vi "trasmision-datos-python-to-Labview.vi"() -> ()   [LabVIEW 2024]
panel:
  in  "trasmitir_START":bool
  in  "Server Closed":string="The server VI closed the connection."
  in  "Stop":bool
  out "Biosignal Graph":dbl[](graph)
  out "*(type *) &x":dbl[](array[numeric])
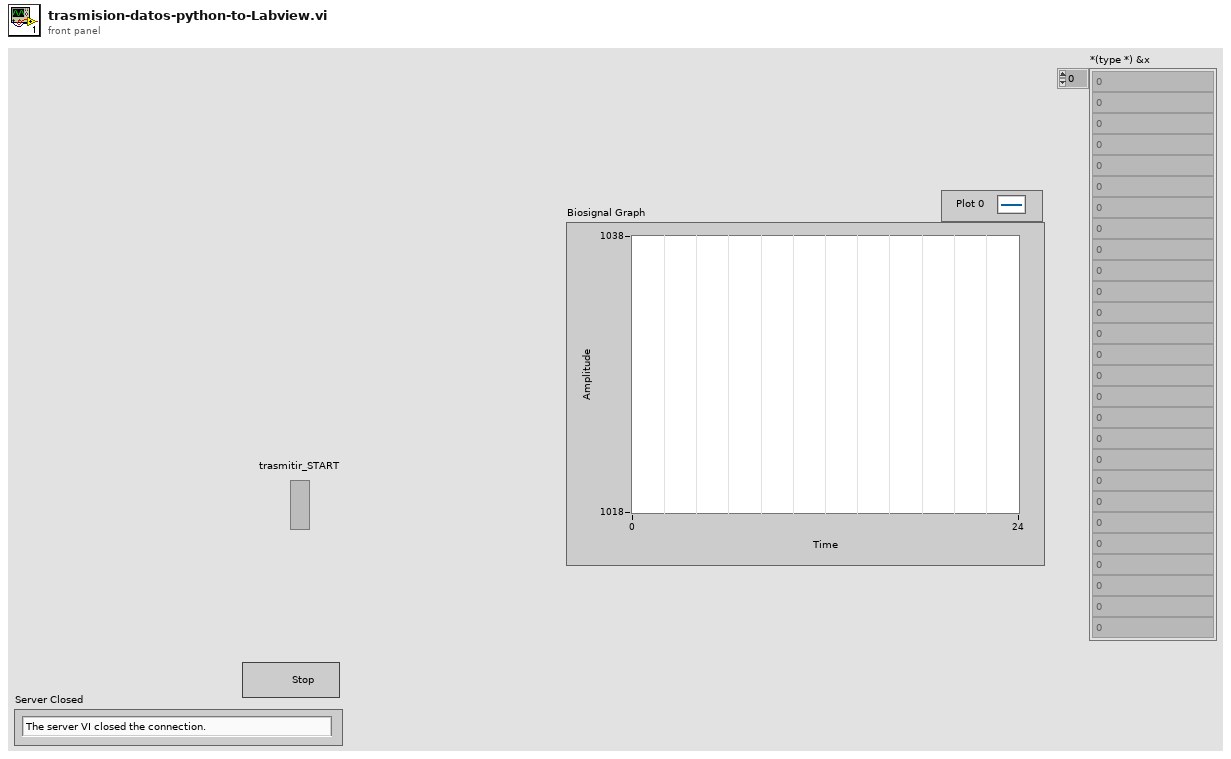
[diagram p1: front panel]
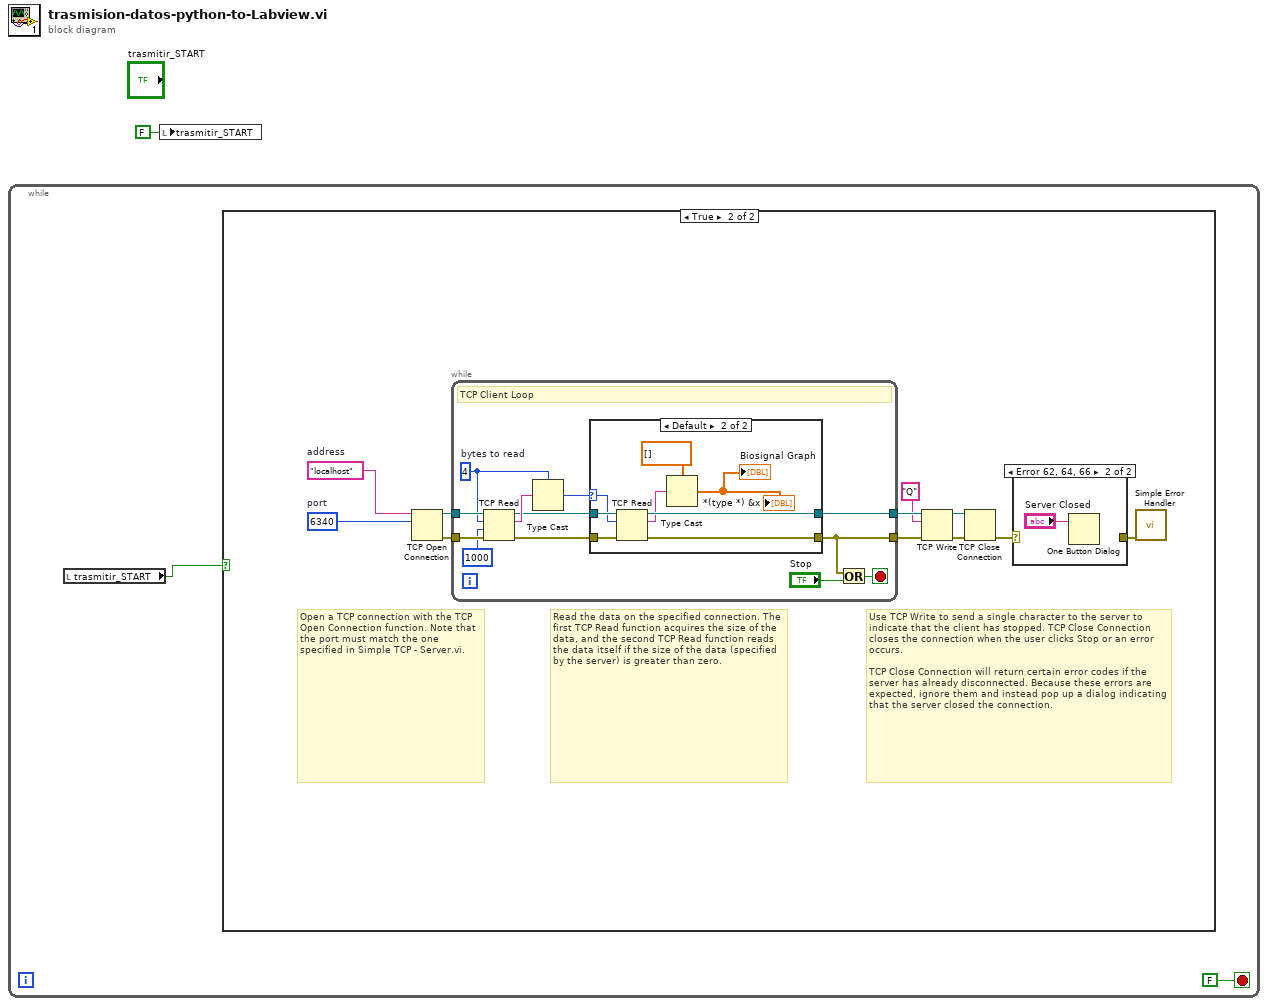
[diagram p0: block diagram]
diagram:
  n1 = while {
    stop <- FALSE stop-if-true
    n2 = local read "trasmitir_START"() -> (w3:bool)
    n3 = case shown="True" w3 {
      frame False {
      }
      frame True {
        w4 = u16 6340  # port
        w5 = "localhost"  # address
        # "Use TCP Write to send a single character to the server to indicate that the client has stopped. TCP Close Connection closes the connection when the user clicks Stop or an error occurs.\n\nTCP Close Connection will return certain error codes if the server has already disconnected. Because these errors are expected, ignore them and instead pop up a dialog indicating that the server closed the connection."
        # "Read the data on the specified connection. The first TCP Read function acquires the size of the data, and the second TCP Read function reads the data itself if the size of the data (specified by the server) is greater than zero."
        # "Open a TCP connection with the TCP Open Connection function. Note that the port must match the one specified in Simple TCP - Server.vi."
        n4 = TCP Open Connection(address=w5, remote port or service name=w4) -> (connection ID=w14:refnum<k5>, error out=w13:errorcluster)  [unwired: 3 in]
        n5 = while {
          tunnel: w13 -> [w24]
          tunnel: w14 -> [w25]
          tunnel: [w20] -> w11
          tunnel: [w19] -> w9
          stop <- w21 stop-if-true
          w23 = 4  # bytes to read
          # "TCP Client Loop"
          n6 = TCP Read(connection ID=w25, bytes to read=w23, error in (no error)=w24, 9:1000 ("timeout ms (25000)")) -> (connection ID out=w27:refnum<k5>, data out=w28:string, error out=w26:errorcluster)  [unwired: 1 in]
          n7 = Type Cast(type=w23, x=w28) -> (*(type *) &x=w18:i32)
          n8 = case shown="Default" w18 {
            selector: w18 -> [_ w31]
            tunnel: w27 -> [w30 w38]
            tunnel: w26 -> [w29 w37]
            tunnel: [w30 w34] -> w20
            tunnel: [w29 w33] -> w19
            frame ..0 {
              # "The server has not written any data"
            }
            frame Default {
              n9 = TCP Read(connection ID=w38, bytes to read=w31, error in (no error)=w37) -> (connection ID out=w34:refnum<k5>, data out=w32:string, error out=w33:errorcluster)  [unwired: 2 in]
              n10 = Type Cast(type=dbl[] [] ("chart"), x=w32) -> (*(type *) &x=→"Biosignal Graph" →"*(type *) &x":dbl[])
            }
          }
          n11 = Or(x=w19, y="Stop") -> (x .or. y?=w21:bool)
        }
        n12 = TCP Write(connection ID=w11, data in="Q", error in (no error)=w9) -> (connection ID out=w12:refnum<k5>, error out=w10:errorcluster)  [unwired: 2 out]
        n13 = TCP Close Connection(connection ID=w12, error in (no error)=w10) -> (error out=w7:errorcluster)  [unwired: 1 in, 1 out]
        n14 = case shown="Error 62, 64, 66" w7 {
          selector: w7 -> [w15 _]
          tunnel: [w15 _] -> w6
          frame #0 {
          }
          frame #1 {
            n15 = One Button Dialog(message="Server Closed") -> ()  [unwired: 1 in, 1 out]
          }
        }
        n16 = call <vilib>:"Simple Error Handler.vi"("error in (no error)"=w6) -> ()  [unwired: 4 in, 5 out]
      }
    }
  }
  n17 = local write "trasmitir_START"(FALSE ("trasmitir_START")) -> ()
